vi "Step Mode - Read Configurations.vi"   [LabVIEW 2014, in "Associated Power Technologies 8500 Series.lvlib"]
uses:
  <instrlib>/Associated Power Technologies 8500 Series/Associated Power Technologies 8500 Series.lvlib
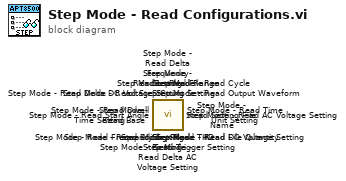
[diagram p0: block diagram]
diagram:
  n1 = call <instrlib>:"Step Mode - Read THD Setting.vi"() -> ()  [unwired: 9 in, 3 out]
  n2 = call <instrlib>:"Step Mode - Read Cycle Setting.vi"() -> ()  [unwired: 9 in, 3 out]
  n3 = call <instrlib>:"Step Mode - Read Dwell Time Setting.vi"() -> ()  [unwired: 9 in, 3 out]
  n4 = call <instrlib>:"Step Mode - Read Time Unit Setting.vi"() -> ()  [unwired: 9 in, 3 out]
  n5 = call <instrlib>:"Step Mode - Read Delta DC Voltage Setting.vi"() -> ()  [unwired: 9 in, 3 out]
  n6 = call <instrlib>:"Step Mode - Read Delta Frequency Setting.vi"() -> ()  [unwired: 9 in, 3 out]
  n7 = call <instrlib>:"Step Mode - Read Delta AC Voltage Setting.vi"() -> ()  [unwired: 9 in, 3 out]
  n8 = call <instrlib>:"Step Mode - Read DC Voltage Setting.vi"() -> ()  [unwired: 9 in, 3 out]
  n9 = call <instrlib>:"Step Mode - Read Frequency Setting.vi"() -> ()  [unwired: 9 in, 3 out]
  n10 = call <instrlib>:"Step Mode - Read AC Voltage Setting.vi"() -> ()  [unwired: 9 in, 3 out]
  n11 = call <instrlib>:"Step Mode - Read Start Angle.vi"() -> ()  [unwired: 9 in, 3 out]
  n12 = call <instrlib>:"Step Mode - Read Output Waveform.vi"() -> ()  [unwired: 9 in, 3 out]
  n13 = call <instrlib>:"Step Mode - Read Range.vi"() -> ()  [unwired: 9 in, 3 out]
  n14 = call <instrlib>:"Step Mode - Read Base.vi"() -> ()  [unwired: 9 in, 3 out]
  n15 = call <instrlib>:"Step Mode - Read Trigger Setting.vi"() -> ()  [unwired: 9 in, 3 out]
  n16 = call <instrlib>:"Step Mode - Read Step Count.vi"() -> ()  [unwired: 9 in, 3 out]
  n17 = call <instrlib>:"Step Mode - Read Setting File Name.vi"() -> ()  [unwired: 9 in, 3 out]
  n18 = call <instrlib>:"Step Mode - Read File Quantity.vi"() -> ()  [unwired: 9 in, 3 out]
  n19 = call <instrlib>:"Step Mode - Read Loaded File.vi"() -> ()  [unwired: 9 in, 3 out]
  n20 = call <instrlib>:"Step Mode - Read Editing File.vi"() -> ()  [unwired: 9 in, 3 out]
